vi "Global Resolution.vi"() -> ()   [LabVIEW 2016]
panel:
  out "Res. in ns":ext=0.031999999999999999999
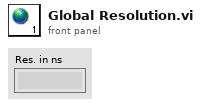
[diagram p1: front panel]
diagram:
